vi "Read Class Data for SubPanel.vi"(8 "error in (no error)":errorcluster, 11 "CIF_UI in":refnum<class "CIF_UI.lvclass">) -> (0 "error out":errorcluster, 2 "Class Data for SubPanel":T1, 3 "CIF_UI out":refnum<class "CIF_UI.lvclass">)   [LabVIEW 2021, in "CIF_UI.lvclass"]
uses:
  CIF_UI.lvclass
  Typedef/Class Data for SubPanel.ctl
  Typedef/Core UI References.ctl
  Typedef/Run Listen Button.ctl
  Typedef/SubPanel Events.ctl
  Typedef/New Connection Plugin Event Data.ctl
  CIF_UI.lvclass/CIF_UI.ctl
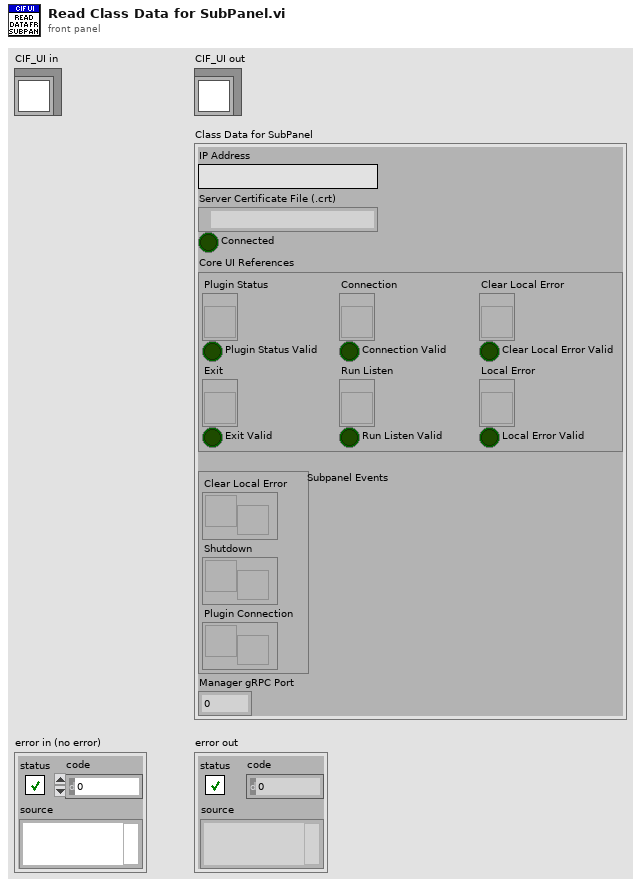
[diagram p1: front panel]
types:
  T1 = typedef "CIF_UI.lvclass/Class Data for SubPanel.ctl" = cluster{"IP Address":string, "Server Certificate File (.crt)":path, "Connected":bool, "Core UI References":T2, "Subpanel Events":T3, "Manager gRPC Port":u16}
  T2 = typedef "CIF_UI.lvclass/Core UI References.ctl" = cluster{"Plugin Status":refnum<vi>, "Plugin Status Valid":bool, "Connection":refnum<vi>, "Connection Valid":bool, "Exit":refnum<vi>, "Exit Valid":bool, "Run Listen":refnum<vi>, "Run Listen Valid":bool, "Clear Local Error":refnum<vi>, "Clear Local Error Valid":bool, "Local Error":refnum<vi>, "Local Error Valid":bool}
  T3 = typedef "CIF_UI.lvclass/SubPanel Events.ctl" = cluster{"Clear Local Error":refnum<user-event>, "Shutdown":refnum<user-event>, "Plugin Connection":refnum<user-event>}
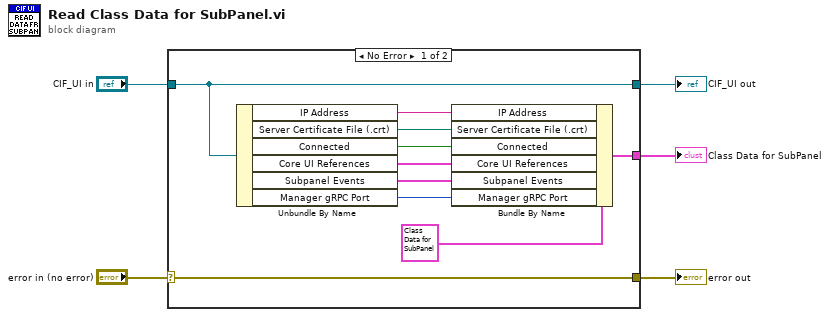
[diagram p0: block diagram]
diagram:
  n1 = case shown="No Error" "error in (no error)" {
    selector: "error in (no error)" -> [w15 w16]
    tunnel: [w15 w16] -> w4
    tunnel: [w14 w17] -> w2
    tunnel: "CIF_UI in" -> [w14 w17]
    tunnel: [w7 _] -> w1
    frame No Error {
      n2 = Unbundle By Name(w14) -> ("IP Address"=w12:string, "Server Certificate File (.crt)"=w8:path, "Connected"=w9:bool, "Core UI References"=w10:T2, "Subpanel Events"=w11:T3, "Manager gRPC Port"=w6:u16)
      n3 = Bundle By Name(cluster=T1 {"IP Address"="", "Server Certificate File (.crt)"=path "", "Connected"=FALSE, "Core UI References"={"Plugin Status"=refnum, "Plugin Status Valid"=FALSE, "Connection"=refnum, "Connection Valid"=FALSE, "Exit"=refnum, "Exit Valid"=FALSE, "Run Listen"=refnum, "Run Listen Valid"=FALSE, "Clear Local Error"=refnum, "Clear Local Error Valid"=FALSE, "Local Error"=refnum, "Local Error Valid"=FALSE}, "Subpanel Events"={"Clear Local Error"=refnum, "Shutdown"=refnum, "Plugin Connection"=refnum}, "Manager gRPC Port"=0} ("Class Data for SubPanel"), "IP Address"=w12, "Server Certificate File (.crt)"=w8, "Connected"=w9, "Core UI References"=w10, "Subpanel Events"=w11, "Manager gRPC Port"=w6) -> (w7:T1)
    }
    frame Error {
    }
  }
  "error out" <- w4
  "CIF_UI out" <- w2
  "Class Data for SubPanel" <- w1
